vi "cleanUpCamera.vi"(8 "error in (no error)":errorcluster, 11 "WebCam in":refnum<class "WebCam.lvclass">) -> (0 "error out":errorcluster, 3 "WebCam out":refnum<class "WebCam.lvclass">)   [LabVIEW 2019, in "WebCam.lvclass"]
uses:
  WebCam.lvclass
  Camera/Camera.lvclass
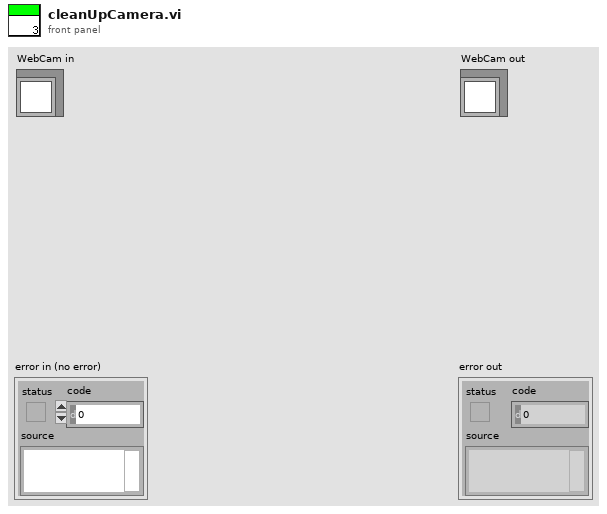
[diagram p1: front panel]
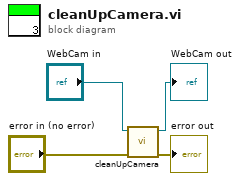
[diagram p0: block diagram]
diagram:
  n1 = call-parent "cleanUpCamera.vi"("error in (no error)"="error in (no error)", "Camera in"="WebCam in") -> ("error out"=→"error out":errorcluster, "Camera out"=→"WebCam out":refnum<class "WebCam.lvclass">)  [unwired: 8 in]
